vi "Set Type Descriptor.vi"(8 "error in (no error)":errorcluster, 10 "Type Descriptor":T1, 11 "Value Editor Base in":refnum<class "Value Editor Base.lvclass">) -> (0 "error out":errorcluster, 3 "Value Editor Base out":refnum<class "Value Editor Base.lvclass">)   [LabVIEW 2020, in "Value Editor Base.lvclass"]
uses:
  Value Editor Base.lvclass
  Type Descriptor.ctl
  Terminal Direction.ctl
  Value Mode.ctl
  Special Terminal.ctl
  Update Type Data.ctl
  Value Editor Base.lvclass/Value Editor Base.ctl
  FlexBlocks.lvlib
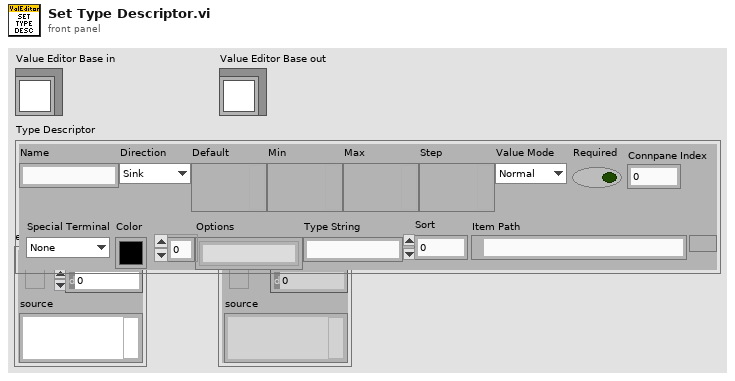
[diagram p1: front panel]
types:
  T1 = typedef "FlexBlocks.lvlib/Type Descriptor.ctl" = cluster{"Name":string, "Direction":T2, "Default":variant, "Min":variant, "Max":variant, "Step":variant, "Value Mode":T3, "Required":bool, "Connpane Index":i32, "Special Terminal":T4, "Color":u32, "Options":string[], "Type String":string, "Sort":i32, "Item Path":path}
  T2 = typedef "FlexBlocks.lvlib/Terminal Direction.ctl" = enum16{"Sink", "Source"}
  T3 = typedef "FlexBlocks.lvlib/Value Mode.ctl" = enum16{"Normal", "Range", "Select"}
  T4 = typedef "FlexBlocks.lvlib/Special Terminal.ctl" = enum16{"None", "Action", "Init", "Tag", "State in", "State out", "Error"}
  T5 = typedef "Value Editor Base.lvclass/Update Type Data.ctl" = cluster{"Type":T1}
  T6 = typedef "Value Editor Base.lvclass/Ref Data.ctl" = cluster{"Type Descriptor":T1, "Terminal Mode":T7, "Value":variant}
  T7 = typedef "FlexBlocks.lvlib/Terminal Mode.ctl" = enum16{"Channel", "Config", "Value", "Control Ref"}
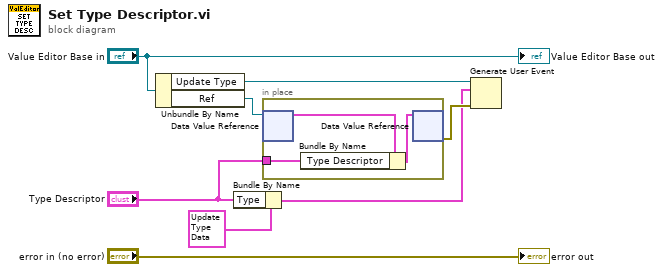
[diagram p0: block diagram]
diagram:
  n1 = Unbundle By Name("Value Editor Base in") -> ("Update Type"=w3:refnum<user-event>, "Ref"=w7:refnum<data-value>)
  n2 = Bundle By Name(cluster=T5 {"Type"={"Name"="", "Direction"=enum."Sink", "Default"=variant, "Min"=variant, "Max"=variant, "Step"=variant, "Value Mode"=enum."Normal", "Required"=FALSE, "Connpane Index"=0, "Special Terminal"=enum."None", "Color"=0, "Options"=[], "Type String"="", "Sort"=0, "Item Path"=path ""}} ("Update Type Data"), "Type"="Type Descriptor") -> (w1:T5)
  n3 = in-place {
    in-place-border: "Type Descriptor" -> [w9]
    n4 = in-place-dvr #1(w7) -> (w11:T6)  [unwired: 1 out]
    n5 = Bundle By Name(cluster=w11, "Type Descriptor"=w9) -> (w10:T6)
    n6 = in-place-dvr #1(w10) -> (w2:errorcluster)  [unwired: 1 out]
  }
  n7 = Generate User Event(user event=w3, event data cluster=w1, error in=w2) -> ()  [unwired: 1 in, 2 out]
  "error out" <- "error in (no error)"
  "Value Editor Base out" <- "Value Editor Base in"
